vi "Init.vi"(8 "error in (no error)":errorcluster, 10 "Team":refnum<class "Team.lvclass">) -> (0 "error out":errorcluster, 3 "Team Dashboard Panel out":refnum<class "Team Dashboard Panel.lvclass">)   [LabVIEW 2020, in "SB App.lvlib" / "Team Dashboard Panel.lvclass"]
uses:
  Team Dashboard Panel.lvclass
  SquareBattle/Team/Team.lvclass
  Team Dashboard Panel.lvclass/Team Dashboard Panel.ctl
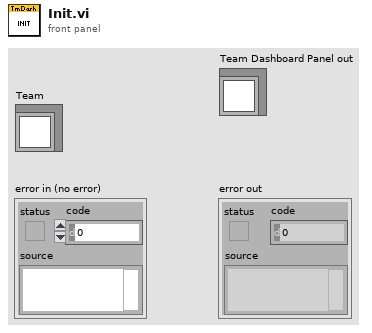
[diagram p1: front panel]
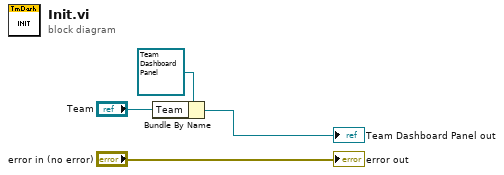
[diagram p0: block diagram]
diagram:
  n1 = Bundle By Name(cluster=refnum<class "Team Dashboard Panel.lvclass"> refnum ("Team Dashboard Panel in"), "Team"="Team") -> (→"Team Dashboard Panel out":refnum<class "Team Dashboard Panel.lvclass">)
  "error out" <- "error in (no error)"
